vi "Handle_Layout_Options.vi"(8 "error in (no error)":errorcluster, 10 "layout options":T1={"orientation (unchanged)"=0, "panel scaling for page (unchanged)"=0, "margins"={"override VI margins (false)"=FALSE, "margins (1.00)"={"top"=1.0, "left"=1.0, "right"=1.0, "bottom"=1.0}, "measurement system (default)"=0}, "printer options"={"destination printer name (current)"="", "printing method (unchanged)"=0, "color or monochrome (unchanged)"=0}, "page header options"={"page headers (unchanged)"=0, "page header content options"={"Include VI Name"=TRUE, "Include VI Path"=TRUE, "Include Last Modification Date"=TRUE, "Include Date Printed"=TRUE, "Include Page Number"=TRUE, "Include VI Icon"=TRUE}}} {"page header options"."page headers (unchanged)" items=["Unchanged", "Include page headers", "Do not include page headers"]; "printer options"."color or monochrome (unchanged)" items=["Unchanged", "Color/grayscale", "Monochrome"]; "printer options"."printing method (unchanged)" items=["Unchanged", "Standard", "PostScript", "Bitmap"]; "panel scaling for page (unchanged)" items=["Unchanged", "No Scaling", "Scale front panel to fit"]; "orientation (unchanged)" items=["Unchanged", "portrait", "landscape"]; "margins"."measurement system (default)" items=["Default", "US", "Metric"]; "margins"."margins (1.00)"."right" format="%.2f"; "margins"."margins (1.00)"."bottom" format="%.2f"; "margins"."margins (1.00)"."top" format="%.2f"; "margins"."margins (1.00)"."left" format="%.2f"}, 11 "VI Refnum":refnum<vi>) -> (0 "error out":errorcluster, 2 "previous layout options":T1={"orientation (unchanged)"=0, "panel scaling for page (unchanged)"=0, "margins"={"override VI margins (false)"=FALSE, "margins (1.00)"={"top"=1.0, "left"=1.0, "right"=1.0, "bottom"=1.0}, "measurement system (default)"=0}, "printer options"={"destination printer name (current)"="", "printing method (unchanged)"=0, "color or monochrome (unchanged)"=0}, "page header options"={"page headers (unchanged)"=0, "page header content options"={"Include VI Name"=TRUE, "Include VI Path"=TRUE, "Include Last Modification Date"=TRUE, "Include Date Printed"=TRUE, "Include Page Number"=TRUE, "Include VI Icon"=TRUE}}} {"page header options"."page headers (unchanged)" items=["Unchanged", "Include page headers", "Do not include page headers"]; "printer options"."color or monochrome (unchanged)" items=["Unchanged", "Color/grayscale", "Monochrome"]; "printer options"."printing method (unchanged)" items=["Unchanged", "Standard", "PostScript", "Bitmap"]; "panel scaling for page (unchanged)" items=["Unchanged", "No Scaling", "Scale front panel to fit"]; "orientation (unchanged)" items=["Unchanged", "portrait", "landscape"]; "margins"."measurement system (default)" items=["Default", "US", "Metric"]; "margins"."margins (1.00)"."right" format="%.2f"; "margins"."margins (1.00)"."bottom" format="%.2f"; "margins"."margins (1.00)"."top" format="%.2f"; "margins"."margins (1.00)"."left" format="%.2f"}, 3 "VI Refnum out":refnum<vi>)   [LabVIEW 2020, in "NI_ReportGenerationCore.lvlib"]
uses:
  <vilib>/Utility/NIReport.llb/NI_ReportGenerationCore.lvlib
  <vilib>/printing/EasyPrintingControls.llb/layout_options.ctl
  <vilib>/printing/EasyPrintingControls.llb/orientation.ctl
  <vilib>/printing/EasyPrintingControls.llb/panel_scaling_for_page.ctl
  <vilib>/printing/EasyPrintingControls.llb/margins.ctl
  <vilib>/printing/EasyPrintingControls.llb/margin_values.ctl
  <vilib>/printing/EasyPrintingControls.llb/measurement_system.ctl
  <vilib>/printing/EasyPrintingControls.llb/printer_options.ctl
  <vilib>/printing/EasyPrintingControls.llb/printing_method.ctl
  <vilib>/printing/EasyPrintingControls.llb/color_or_monochrome.ctl
  <vilib>/printing/EasyPrintingControls.llb/page_header_options.ctl
  <vilib>/printing/EasyPrintingControls.llb/page_headers.ctl
  <vilib>/printing/EasyPrintingControls.llb/page_header_content_options.ctl
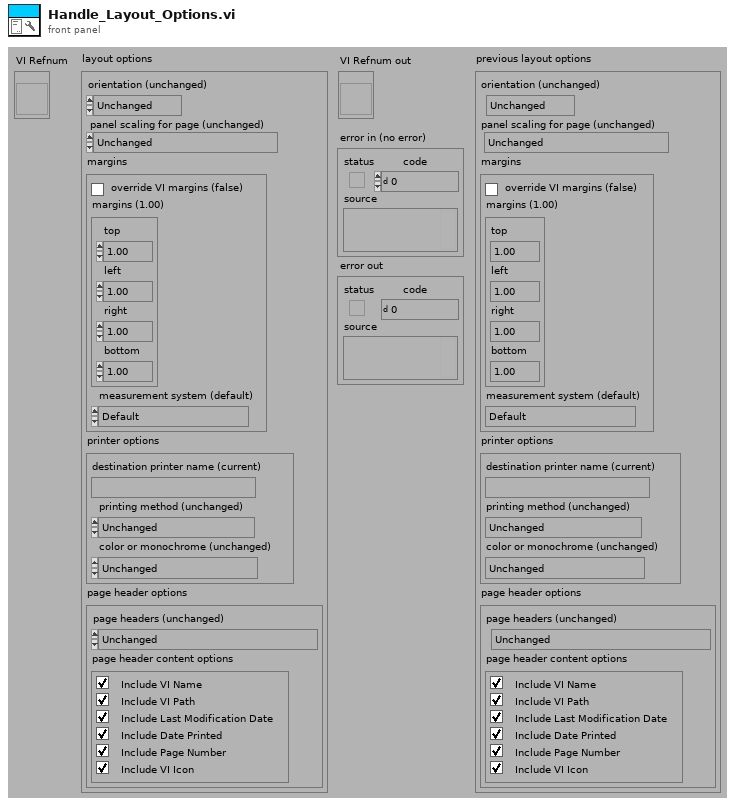
[diagram p1: front panel]
types:
  T1 = typedef "NI_ReportGenerationCore.lvlib/layout_options.ctl" = cluster{"orientation (unchanged)":T2, "panel scaling for page (unchanged)":T3, "margins":T4, "printer options":T7, "page header options":T10}
  T2 = typedef "NI_ReportGenerationCore.lvlib/orientation.ctl" = u16
  T3 = typedef "NI_ReportGenerationCore.lvlib/panel_scaling_for_page.ctl" = u16
  T4 = typedef "NI_ReportGenerationCore.lvlib/margins.ctl" = cluster{"override VI margins (false)":bool, "margins (1.00)":T5, "measurement system (default)":T6}
  T5 = typedef "NI_ReportGenerationCore.lvlib/margin_values.ctl" = cluster{"top":dbl, "left":dbl, "right":dbl, "bottom":dbl}
  T6 = typedef "NI_ReportGenerationCore.lvlib/measurement_system.ctl" = u16
  T7 = typedef "NI_ReportGenerationCore.lvlib/printer_options.ctl" = cluster{"destination printer name (current)":string, "printing method (unchanged)":T8, "color or monochrome (unchanged)":T9}
  T8 = typedef "NI_ReportGenerationCore.lvlib/printing_method.ctl" = u16
  T9 = typedef "NI_ReportGenerationCore.lvlib/color_or_monochrome.ctl" = u16
  T10 = typedef "NI_ReportGenerationCore.lvlib/page_header_options.ctl" = cluster{"page headers (unchanged)":T11, "page header content options":T12}
  T11 = typedef "NI_ReportGenerationCore.lvlib/page_headers.ctl" = u16
  T12 = typedef "NI_ReportGenerationCore.lvlib/page_header_content_options.ctl" = cluster{"Include VI Name":bool, "Include VI Path":bool, "Include Last Modification Date":bool, "Include Date Printed":bool, "Include Page Number":bool, "Include VI Icon":bool}
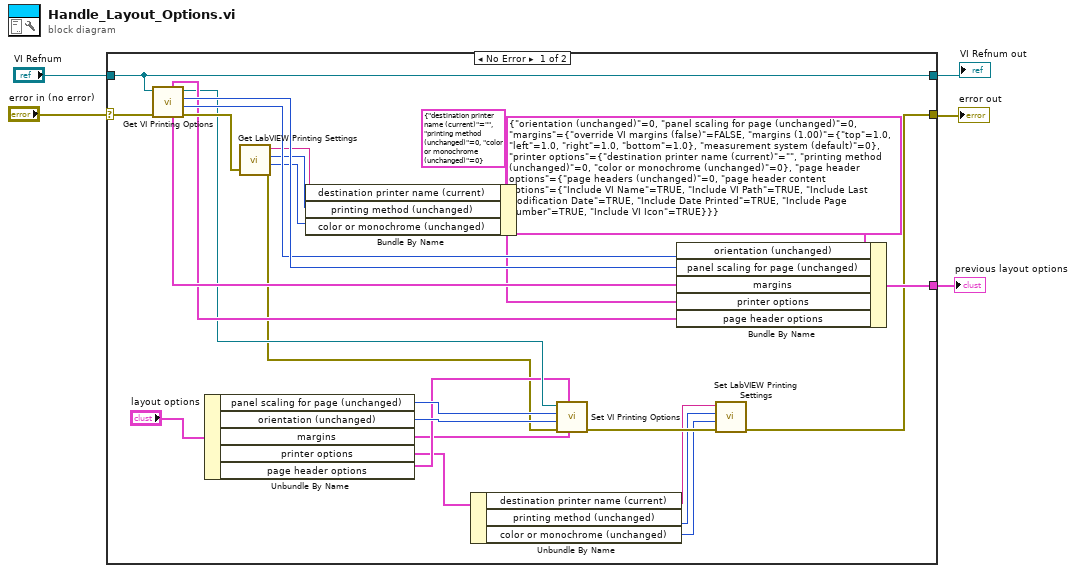
[diagram p0: block diagram]
diagram:
  n1 = case shown="No Error" "error in (no error)" {
    selector: "error in (no error)" -> [w31 w34]
    tunnel: [w7 w34] -> w4
    tunnel: [w32 w33] -> w2
    tunnel: "VI Refnum" -> [w32 w33]
    tunnel: [w19 _] -> w1
    frame No Error {
      n2 = call <vilib>:"Get VI Printing Options.vi"("error in (no error)"=w31, "VI Refnum"=w32) -> ("error out"=w30:errorcluster, "orientation (unchanged)"=w28:T2, "panel scaling for page (unchanged)"=w29:T3, "VI Refnum out"=w17:refnum<vi>, "margins"=w27:T4, "page header options"=w20:T10)  [unwired: 4 in]
      n3 = Unbundle By Name("layout options") -> ("panel scaling for page (unchanged)"=w15:T3, "orientation (unchanged)"=w14:T2, "margins"=w12:T4, "printer options"=w11:T7, "page header options"=w13:T10)
      n4 = call <vilib>:"Get LabVIEW Printing Settings.vi"("error in (no error)"=w30) -> ("error out"=w6:errorcluster, "color or monochrome"=w25:T9, "printing method"=w24:T8, "default printer name"=w26:string)  [unwired: 7 in]
      n5 = Bundle By Name(cluster=T7 {"destination printer name (current)"="", "printing method (unchanged)"=0, "color or monochrome (unchanged)"=0} ("printer options"), "destination printer name (current)"=w26, "printing method (unchanged)"=w24, "color or monochrome (unchanged)"=w25) -> (w23:T7)
      n6 = Unbundle By Name(w11) -> ("destination printer name (current)"=w10:string, "printing method (unchanged)"=w9:T8, "color or monochrome (unchanged)"=w8:T9)
      n7 = call <vilib>:"Set VI Printing Options.vi"("margins"=w12, "page header options"=w13, "error in (no error)"=w6, "orientation (unchanged)"=w14, "panel scaling for page (unchanged)"=w15, "VI Refnum"=w17) -> ("error out"=w16:errorcluster)  [unwired: 4 in, 1 out]
      n8 = Bundle By Name(cluster=T1 {"orientation (unchanged)"=0, "panel scaling for page (unchanged)"=0, "margins"={"override VI margins (false)"=FALSE, "margins (1.00)"={"top"=1.0, "left"=1.0, "right"=1.0, "bottom"=1.0}, "measurement system (default)"=0}, "printer options"={"destination printer name (current)"="", "printing method (unchanged)"=0, "color or monochrome (unchanged)"=0}, "page header options"={"page headers (unchanged)"=0, "page header content options"={"Include VI Name"=TRUE, "Include VI Path"=TRUE, "Include Last Modification Date"=TRUE, "Include Date Printed"=TRUE, "Include Page Number"=TRUE, "Include VI Icon"=TRUE}}} ("previous layout options"), "orientation (unchanged)"=w28, "panel scaling for page (unchanged)"=w29, "margins"=w27, "printer options"=w23, "page header options"=w20) -> (w19:T1)
      n9 = call <vilib>:"Set LabVIEW Printing Settings.vi"("error in (no error)"=w16, "color or monochrome"=w8, "printing method"=w9, "default printer name"=w10) -> ("error out"=w7:errorcluster)  [unwired: 7 in]
    }
    frame Error {
    }
  }
  "error out" <- w4
  "VI Refnum out" <- w2
  "previous layout options" <- w1
